vi "NIIE_Layer_GraphicManipulation.vi"(7 "Radio Buttons":T2=enum."Ellipse", 8 "Error":errorcluster, 10 "Position":T1, 11 "Layer.lvclass":refnum<class "Layer.lvclass">) -> (0 "Error Out":errorcluster, 2 "Operation Processed? Out":bool, 3 "Layer.lvclass Out":refnum<class "Layer.lvclass">)   [LabVIEW 2021]
uses:
  vi.lib/LabVIEW Icon API/lv_icon/Classes/Layer/Layer.lvclass
  MB CORE/TypeDefs/Cluster_Button Draw Tools.ctl
  MB CORE/TypeDefs/Bool_Draw Tool.ctl
  MB CORE/TypeDefs/Bool_Line Tool.ctl
  MB CORE/TypeDefs/Bool_ColorExtractor Tool.ctl
  MB CORE/TypeDefs/Bool_Fill Tool.ctl
  MB CORE/TypeDefs/Bool_IERect Tool.ctl
  MB CORE/TypeDefs/Bool_FRect Tool.ctl
  MB CORE/TypeDefs/Bool_Circle Tool.ctl
  MB CORE/TypeDefs/Bool_FillCircle Tool.ctl
  MB CORE/TypeDefs/Bool_Eraser Tool.ctl
  MB CORE/TypeDefs/Bool_Text Tool.ctl
  MB CORE/TypeDefs/Bool_Selection Tool.ctl
  MB CORE/TypeDefs/Bool_Move Tool.ctl
  <vilib>/Utility/miscctls.llb/LVPositionTypeDef.ctl
  vi.lib/LabVIEW Icon API/lv_icon/lv_icon.lvlib
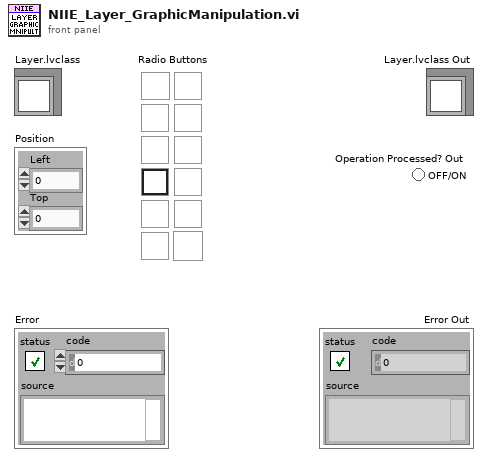
[diagram p1: front panel]
types:
  T1 = typedef "LVPositionTypeDef.ctl" = cluster{"Left":i32, "Top":i32}
  T2 = typedef "Cluster_Button Draw Tools.ctl" = enum32{"Pencil", "Line", "Dropper", "Fill", "Rectangle", "Filled Rectangle", "Ellipse", "Filled Ellipse", "Eraser", "Text", "Select", "Move"}
  T3 = typedef "Cluster_Layer Data.ctl" = cluster{"LayerIcon":picture, "LayerName":string, "Opacity":u8, "Visibility?":bool}
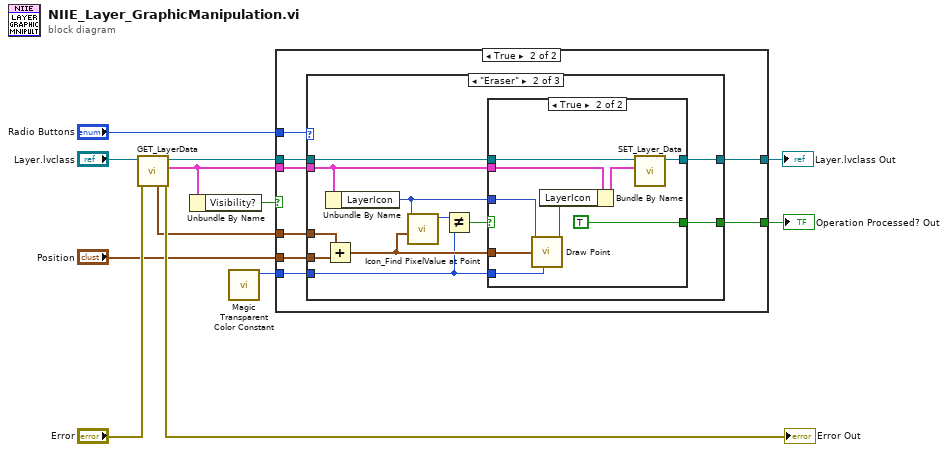
[diagram p0: block diagram]
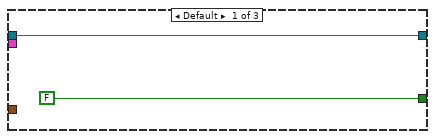
[diagram p3: hidden frame]
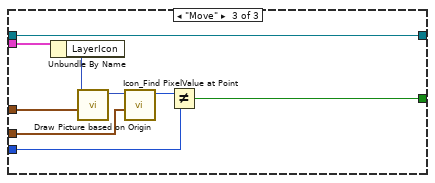
[diagram p5: hidden frame]
diagram:
  n1 = call-dynamic "GET_LayerData.vi"("error in (no error)"="Error", "Layer.lvclass in"="Layer.lvclass") -> ("error out"=→"Error Out":errorcluster, "Data"=w9:T3, "Layer.lvclass out"=w10:refnum<class "Layer.lvclass">, "Origin"=w7:T1)  [unwired: 6 out]
  n2 = Unbundle By Name(w9) -> ("Visibility?"=w5:bool)
  n3 = call "Magic Transparent Color Constant.vi"() -> ("Magic transparent color constant"=w1:u32)  [unwired: 11 out]
  n4 = case shown="True" w5 {
    tunnel: w7 -> [_ w21]
    tunnel: "Position" -> [_ w20]
    tunnel: w9 -> [_ w19]
    tunnel: w10 -> [w13 w18]
    tunnel: [w13 w17] -> w11
    tunnel: "Radio Buttons" -> [_ w16]
    tunnel: [_ w15] -> w3
    tunnel: w1 -> [_ w14]
    frame False {
    }
    frame True {
      n5 = case shown="\"Eraser\"" w16 {
        tunnel: w21 -> [_ w29 w53]
        tunnel: w20 -> [_ w28 w52]
        tunnel: w19 -> [_ w26 w48]
        tunnel: w18 -> [w23 w32 w50]
        tunnel: [w23 w31 w50] -> w17
        tunnel: [FALSE w30 w49] -> w15
        tunnel: w14 -> [_ w24 w46]
        frame Default {
        }
        frame "Eraser" {
          n6 = Add(x=w29, y=w28) -> (x+y=w27:T1)
          n7 = Unbundle By Name(w26) -> ("LayerIcon"=w25:picture)
          n8 = call "Icon_Find PixelValue at Point.vi"("Point"=w27, "Picture"=w25) -> ("Color Box Out"=w34:u32)  [unwired: 9 out]
          n9 = Not Equal?(x=w34, y=w24) -> (x != y?=w33:bool)
          n10 = case shown="True" w33 {
            selector: w33 -> [w35 _]
            tunnel: w24 -> [_ w44]
            tunnel: w27 -> [_ w43]
            tunnel: w26 -> [_ w42]
            tunnel: w25 -> [_ w41]
            tunnel: w32 -> [w36 w39]
            tunnel: [w36 w38] -> w31
            tunnel: [w35 TRUE] -> w30
            frame False {
            }
            frame True {
              n11 = call <vilib>:"Draw Point.vi"("picture"=w41, "point(x,y)"=w43, "color(black)"=w44) -> ("new picture"=w45:picture)  [unwired: 1 in, 5 out]
              n12 = Bundle By Name(cluster=w42, "LayerIcon"=w45) -> (w40:T3)
              n13 = call-dynamic "SET_Layer_Data.vi"("Data"=w40, "Layer.lvclass in"=w39) -> ("Layer.lvclass out"=w38:refnum<class "Layer.lvclass">)  [unwired: 2 in, 7 out]
            }
          }
        }
        frame "Move" {
          n14 = Unbundle By Name(w48) -> ("LayerIcon"=w47:picture)
          n15 = call "Draw Picture based on Origin.vi"("Origin"=w53, "LayerIcon in"=w47) -> ("LayerIcon out"=w51:picture)  [unwired: 1 in, 8 out]
          n16 = call "Icon_Find PixelValue at Point.vi"("Point"=w52, "Picture"=w51) -> ("Color Box Out"=w54:u32)  [unwired: 9 out]
          n17 = Not Equal?(x=w54, y=w46) -> (x != y?=w49:bool)
        }
      }
    }
  }
  "Layer.lvclass Out" <- w11
  "Operation Processed? Out" <- w3
